vi "Move Object.vi"(7 "Direction":enum16{"Up", "Down", "Left", "Right"}(ring)=enum."Right", 8 "error in (no error)":errorcluster, 10 "Frame Bounds":T1, 11 "Object to Move":refnum<vi>) -> (0 "error out":errorcluster, 3 "number of pixels to move":u32)   [LabVIEW 2011]
uses:
  <vilib>/Utility/miscctls.llb/LVRectTypeDef.ctl
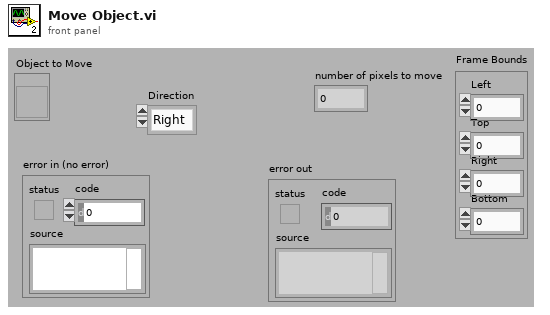
[diagram p1: front panel]
types:
  T1 = typedef "LVRectTypeDef.ctl" = cluster{"Left":i16, "Top":i16, "Right":i16, "Bottom":i16}
  T2 = typedef "LVPositionTypeDef.ctl" = cluster{"Left":i32, "Top":i32}
  T3 = typedef "LVBoundsTypeDef.ctl" = cluster{"Width":u32, "Height":u32}
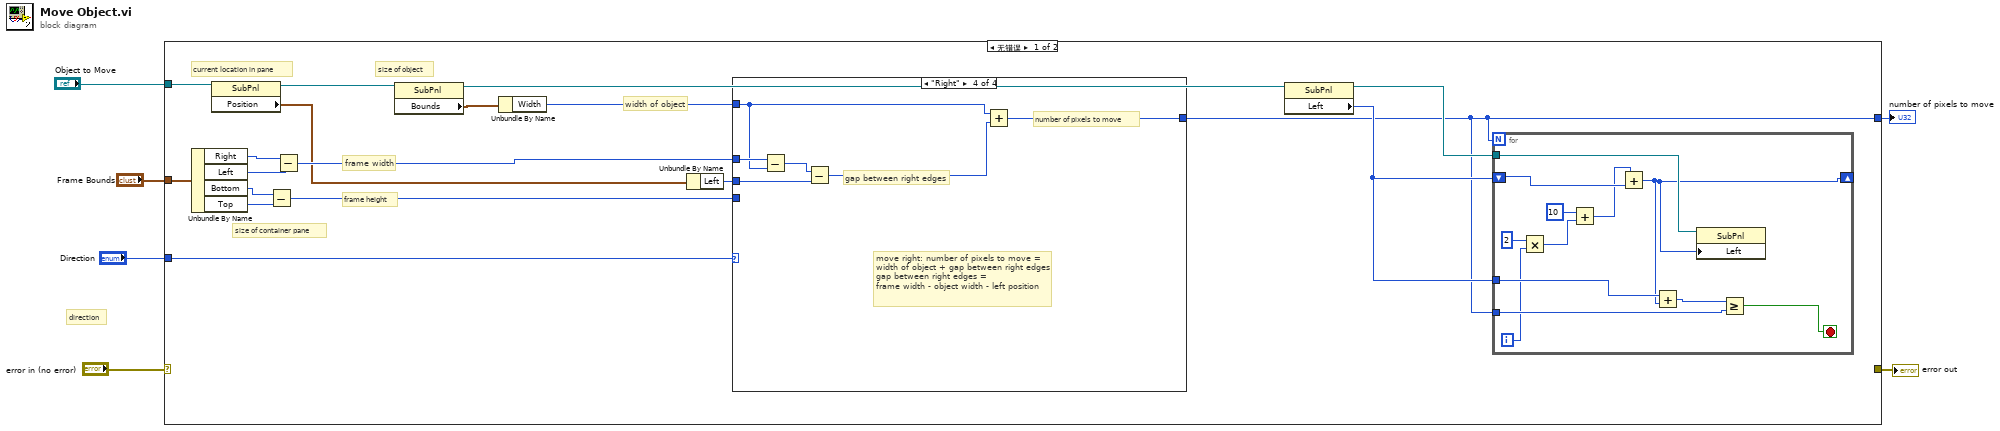
[diagram p0: block diagram]
diagram:
  # "direction"
  n1 = case shown="无错误" "error in (no error)" {
    selector: "error in (no error)" -> [_ w43]
    tunnel: [_ w43] -> w6
    tunnel: "Object to Move" -> [w24 _]
    tunnel: "Direction" -> [w18 _]
    tunnel: "Frame Bounds" -> [w20 _]
    tunnel: [w7 _] -> w2
    frame No Error {
      # "frame height"
      # "frame width"
      # "width of object"
      # "size of object"
      # "size of container pane"
      # "current location in pane"
      n2 = Unbundle By Name(w20) -> ("Right"=w23:i16, "Left"=w13:i16, "Bottom"=w22:i16, "Top"=w21:i16)
      n3 = property class="SubPnl"(reference=w24) -> (reference out=w19:refnum<vi>, "Position"=w12:T2)  [unwired: 1 in, 1 out]
      n4 = Subtract(x=w22, y=w21) -> (x-y=w14:i16)
      n5 = Subtract(x=w23, y=w13) -> (x-y=w15:i16)
      n6 = property class="SubPnl"(reference=w19) -> (reference out=w10:refnum<vi>, "Bounds"=w17:T3)  [unwired: 1 in, 1 out]
      n7 = Unbundle By Name(w17) -> ("Width"=w16:u32)
      n8 = Unbundle By Name(w12) -> ("Left"=w11:i32)
      n9 = case shown="\"Right\"" w18 {
        tunnel: w16 -> [_ _ _ w39]
        tunnel: w15 -> [_ _ _ w42]
        tunnel: w14 -> [_ _ _ _]
        tunnel: w11 -> [_ _ _ w40]
        tunnel: [_ _ _ w37] -> w7
        frame "Up", Default {
        }
        frame "Down" {
        }
        frame "Left" {
        }
        frame "Right" {
          # "number of pixels to move"
          # "gap between right edges"
          # "move right: number of pixels to move = \nwidth of object + gap between right edges\ngap between right edges = \nframe width - object width - left position"
          n10 = Subtract(x=w42, y=w39) -> (x-y=w41:u32)
          n11 = Subtract(x=w41, y=w40) -> (x-y=w38:u32)
          n12 = Add(x=w39, y=w38) -> (x+y=w37:u32)
        }
      }
      n13 = property class="SubPnl"(reference=w10) -> (reference out=w9:refnum<vi>, "Left"=w8:i32)  [unwired: 1 in, 1 out]
      n14 = for {
        N: w7 -> [_]
        tunnel: w9 -> [w36]
        shift-right: [w33] -> _
        shift-left: w8 -> [w35]
        tunnel: w8 -> [w34]
        tunnel: w7 -> [w31]
        i -> [w29]
        stop <- w30 stop-if-true
        n15 = Multiply(x=2, y=w29) -> (x*y=w27:i32)
        n16 = Add(x=10, y=w27) -> (x+y=w26:i32)
        n17 = Add(x=w26, y=w35) -> (x+y=w33:i32)
        n18 = Add(x=w34, y=w33) -> (x+y=w32:i32)
        n19 = property class="SubPnl"(reference=w36, "Left"=w33) -> ()  [unwired: 1 in, 2 out]
        n20 = Greater Or Equal?(x=w32, y=w31) -> (x >= y?=w30:bool)
      }
    }
    frame Error {
    }
  }
  "error out" <- w6
  "number of pixels to move" <- w2
